vi "Save McP CounterPos.dat.vi"(1 "Error Code (0: No Error)":i32, 2 "McP Counter Position Path":path, 3 "Last Calibration Date":string="Thursday, January 7, 1904 11:42 AM\r", 4 "Set Method":u16(ring)=3 items=["Moving", "Calibration", "Key in", "Initialization"], 5 "McP Stepper Position":i32, 6 "McP Counter Position":dbl=2874.99953 format="%.5f") -> (0 "Written content":string="#   McPherson 789A-3 Counter Position:    2874.99953\r#   McPherson 789A-3 STEPPER Position:   0\r#   Error Code:   0   @DATE:   Tuesday, February 22, 2011 1:25 PM\r#   Set by Initialization\r#   Last Calibration Date:  Thursday, January 7, 1904 11:42 AM\r\r\rLast FIVE transactions:\r\r#   McPherson 789A-3 Counter Position:    2874.99953\r#   McPherson 789A-3 STEPPER Position:   0\r#   Error Code:   9240   @DATE:   Tuesday, February 22, 2011 11:28 AM\r#   Set by Moving\r#   Last Calibration Date:  Thursday, January 7, 1904 11:42 AM\r\r\r#   McPherson 789A-3 Counter Position:    2874.99953\r#   McPherson 789A-3 STEPPER Position:   78125\r#   Error Code:   0   @DATE:   Saturday, August 5, 2006 5:12 PM\r#   Set by Moving\r#   Last Calibration Date:  Thursday, January 7, 1904 11:42 AM\r\r\r#   McPherson 789A-3 Counter Position:    2624.99953\r#   McPherson 789A-3 STEPPER Position:   15625\r#   Error Code:   0   @DATE:   Saturday, August 5, 2006 5:12 PM\r#   Set by Moving\r#   Last Calibration Date:  Thursday, January 7, 1904 11:42 AM\r\r\r#   McPherson 789A-3 Counter Position:    2499.99953\r#   McPherson 789A-3 STEPPER Position:   -15625\r#   Error Code:   0   @DATE:   Saturday, August 5, 2006 5:11 PM\r#   Set by Moving\r#   Last Calibration Date:  Thursday, January 7, 1904 11:42 AM\r\r\r#   McPherson 789A-3 Counter Position:    2249.99953\r#   McPherson 789A-3 STEPPER Position:   -78125\r#   Error Code:   0   @DATE:   Saturday, August 5, 2006 5:11 PM\r#   Set by Moving\r#   Last Calibration Date:  Thursday, January 7, 1904 11:42 AM\r")   [LabVIEW 2025]
doc: "Author: Scott Hannahs <sth@magnet.fsu.edu>\n\nThis software is licensed for use under the “MIT License\"\nCopyright (c) 2025 Scott Hannahs, sth@sth@magnet.sthnet.net\n\nPermission is hereby granted, free of charge, to any person obtaining a copy of this software and associated documentation files (the \"Software\"), to deal in the Software without restriction, including without limitation the rights to use, copy, modify, merge, publish, distribute, sublicense, and/or sell copies of the Software, and to permit persons to whom the Software is furnished to do so, subject to the following conditions: The above copyright notice and this permission notice shall be included in all copies or substantial portions of the Software.\n\nTHE SOFTWARE IS PROVIDED \"AS IS\", WITHOUT WARRANTY OF ANY KIND, EXPRESS OR IMPLIED, INCLUDING BUT NOT LIMITED TO THE WARRANTIES OF MERCHANTABILITY, FITNESS FOR A PARTICULAR PURPOSE AND NONINFRINGEMENT. IN NO EVENT SHALL THE AUTHORS OR COPYRIGHT HOLDERS BE LIABLE FOR ANY CLAIM, DAMAGES OR OTHER LIABILITY, WHETHER IN AN ACTION OF CONTRACT, TORT OR OTHERWISE, ARISING FROM, OUT OF OR IN CONNECTION WITH THE SOFTWARE OR THE USE OR OTHER DEALINGS IN THE SOFTWARE."
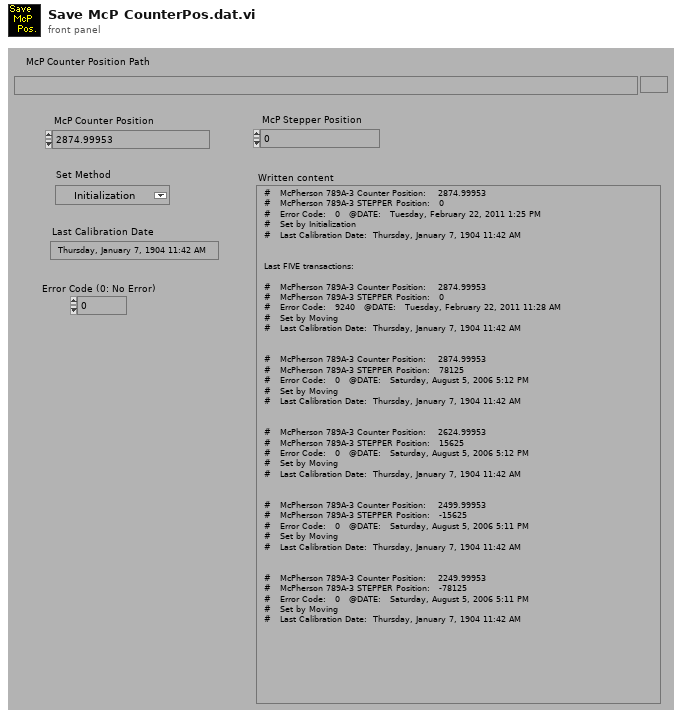
[diagram p1: front panel]
types:
  T1 = enum16{"open", "open or create", "create or replace", "create"}
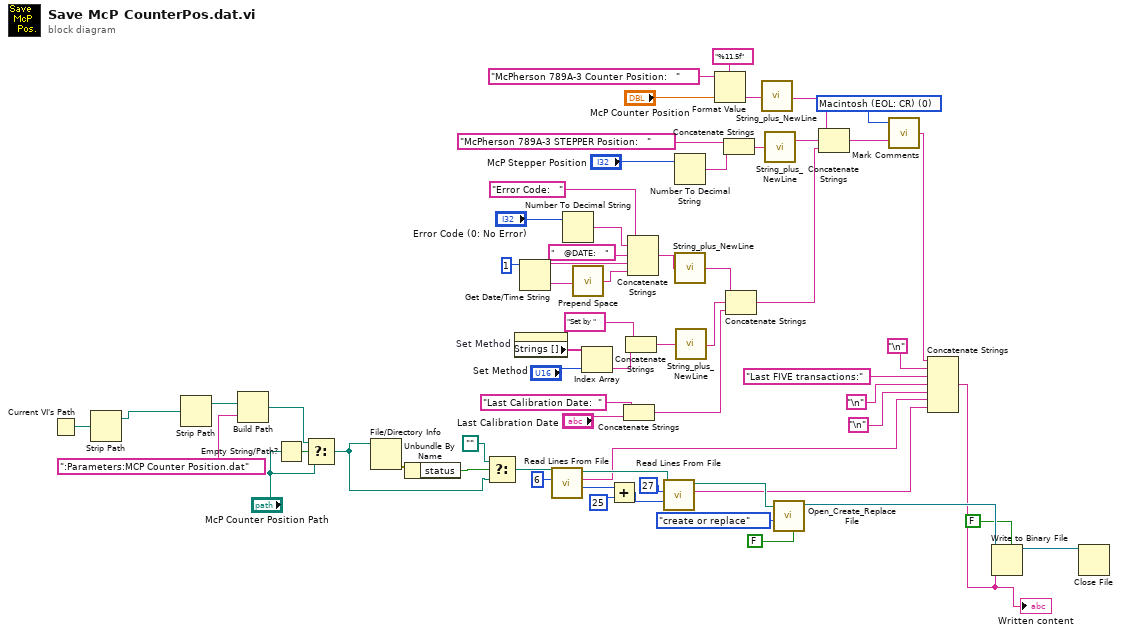
[diagram p0: block diagram]
diagram:
  w52 = u16 0 items=["Macintosh (EOL: CR)", "Unix (EOL: LF)", "DOS/Windows (EOL: CR+LF)"] ("File Format")
  n1 = Current VI's Path() -> (path=w8:path)
  n2 = Strip Path(path=w8) -> (stripped path=w4:path)  [unwired: 1 out]
  n3 = Strip Path(path=w4) -> (stripped path=w9:path)  [unwired: 1 out]
  n4 = Build Path(base path=w9, name or relative path=":Parameters:MCP Counter Position.dat") -> (appended path=w7:path)
  n5 = Empty String/Path?(string/path="McP Counter Position Path") -> (empty?=w11:bool)
  n6 = Select(t=w7, s=w11, f="McP Counter Position Path") -> (s? t:f=w5:path)
  n7 = File/Directory Info(path=w5) -> (error out=w15:errorcluster)  [unwired: 1 in, 6 out]
  n8 = Unbundle By Name(w15) -> ("status"=w14:bool)
  n9 = Select(t=path "", s=w14, f=w5) -> (s? t:f=w12:path)
  n10 = property on="Set Method" class="Ring (strict)"() -> ("Strings []"=w40:string[])  [unwired: 2 in, 2 out]
  n11 = Get Date/Time String(date format (0)=1) -> (date string=w54:string, time string=w2:string)  [unwired: 2 in]
  n12 = call <vilib>:"Read Lines From File.vi"("file path (dialog if empty)"=w12, "number of lines (all:-1)"=6) -> ("new file path (Not A Path if cancelled)"=w32:path, "line string"=w22:string, "mark after read (chars.)"=w34:i32)  [unwired: 4 in, 1 out]
  n13 = Number To Decimal String(number="Error Code (0: No Error)") -> (decimal integer string=w17:string)  [unwired: 1 in]
  n14 = call "Prepend Space.vi"("Input String"=w2) -> ("Space + Input String"=w1:string)
  n15 = Index Array(array=w40, index="Set Method") -> (element=w39:string)
  n16 = Add(x=w34, y=25) -> (x+y=w31:i32)
  n17 = Concatenate Strings("Last Calibration Date:  ", "Last Calibration Date") -> (w38:string)
  n18 = Concatenate Strings("Set by ", w39) -> (w49:string)
  n19 = Concatenate Strings("Error Code:   ", w17, "   @DATE:   " ("date string"), w54, w1) -> (w51:string)
  n20 = call <vilib>:"Read Lines From File.vi"("file path (dialog if empty)"=w32, "number of lines (all:-1)"=27, "start of read offset (chars.:0)"=w31) -> ("new file path (Not A Path if cancelled)"=w29:path, "line string"=w21:string)  [unwired: 3 in, 2 out]
  n21 = Number To Decimal String(number="McP Stepper Position") -> (decimal integer string=w56:string)  [unwired: 1 in]
  n22 = call "String_plus_NewLine.vi"("Input String"=w51) -> ("Input String +[\\n]"=w45:string)
  n23 = call "String_plus_NewLine.vi"("Input String"=w49) -> ("Input String +[\\n]"=w44:string)
  n24 = Format Value(string ("")="McPherson 789A-3 Counter Position:   ", format string="%11.5f", value (0)="McP Counter Position") -> (output string=w53:string)
  n25 = Concatenate Strings("McPherson 789A-3 STEPPER Position:   ", w56) -> (w48:string)
  n26 = Concatenate Strings(w45, w44, w38) -> (w37:string)
  n27 = call "String_plus_NewLine.vi"("Input String"=w53) -> ("Input String +[\\n]"=w43:string)
  n28 = call "String_plus_NewLine.vi"("Input String"=w48) -> ("Input String +[\\n]"=w42:string)
  n29 = call <vilib>:"Open_Create_Replace File.vi"("advisory dialog? (display:T)"=FALSE, "function (open:0)"=T1."create or replace", "file path"=w29) -> ("refnum"=w28:refnum<file>)  [unwired: 5 in, 3 out]
  n30 = Concatenate Strings(w43, w42, w37) -> (w36:string)
  n31 = call "Mark Comments.vi"("Input String"=w36, "File Format"=w52) -> ("Output String"=w27:string)  [unwired: 1 in]
  n32 = Concatenate Strings(w27, "\n", "Last FIVE transactions:", "\n", "\n", w22, w21) -> (w20:string)
  "Written content" <- w20
  n33 = Write to Binary File(file (use dialog)=w28, data=w20, 5:FALSE ("prepend array or string size? (T)")) -> (refnum out=w60:refnum<file>)  [unwired: 3 in, 2 out]
  n34 = Close File(refnum=w60) -> ()  [unwired: 1 in, 2 out]
